vi "Get All Values from Database.vi"(8 "error in (no error)":errorcluster, 11 "String Database in":refnum<class "String Database.lvclass">=refnum) -> (0 "error out":errorcluster, 1 "Values":string[](array[string]), 2 "Names":string[](array[string]), 3 "String Database out":refnum<class "String Database.lvclass">)   [LabVIEW 2018, in "String Database.lvlib" / "String Database.lvclass"]
uses:
  String Database.lvclass
  String Database.lvclass/String Database.ctl
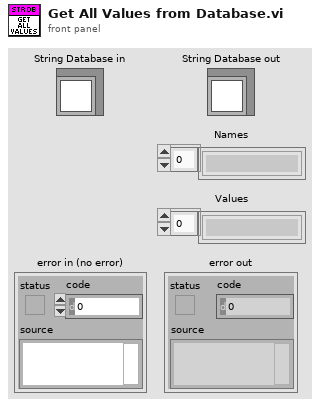
[diagram p1: front panel]
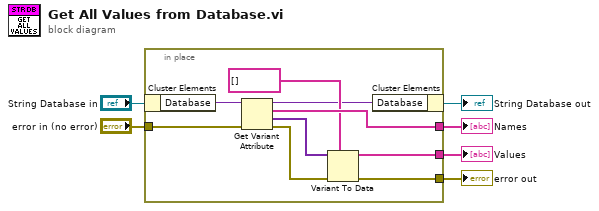
[diagram p0: block diagram]
diagram:
  n1 = in-place {
    in-place-border: "error in (no error)" -> [w15]
    in-place-border: [w14] -> w5
    in-place-border: [w13] -> w4
    in-place-border: [w12] -> w3
    n2 = in-place-cluster #1("String Database in") -> ("Database"=w8:variant)
    n3 = Get Variant Attribute(Variant=w8, error in=w15) -> (duplicate Variant=w7:variant, names=w13:string[], values=w11:variant[], error out=w9:errorcluster)  [unwired: 2 in]
    n4 = Variant To Data(error in=w9, type=string[] [], Variant=w11) -> (data=w12:string[], error out=w14:errorcluster)
    n5 = in-place-cluster #1("Database"=w7) -> (→"String Database out":refnum<class "String Database.lvclass">)
  }
  "error out" <- w5
  "Names" <- w4
  "Values" <- w3
